vi "calc_trans.vi"(0 "Reference":T1, 3 "Input":T2) -> ()   [LabVIEW 2024]
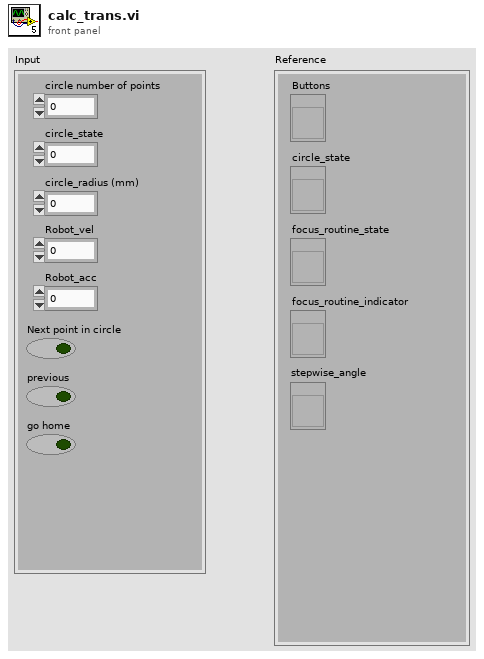
[diagram p1: front panel]
types:
  T1 = cluster{"Buttons":refnum<vi>, "circle_state":refnum<vi>, "focus_routine_state":refnum<vi>, "focus_routine_indicator":refnum<vi>, "stepwise_angle":refnum<vi>}
  T2 = cluster{"circle number of points":i8, "circle_state":i8, "circle_radius (mm)":dbl, "Robot_vel":dbl, "Robot_acc":dbl, "Next point in circle":bool, "previous":bool, "go home":bool}
  T3 = cluster{"Focus routine":bool, "Freedrive mode":bool, "Next point in circle":bool, "previous":bool, "go home":bool}
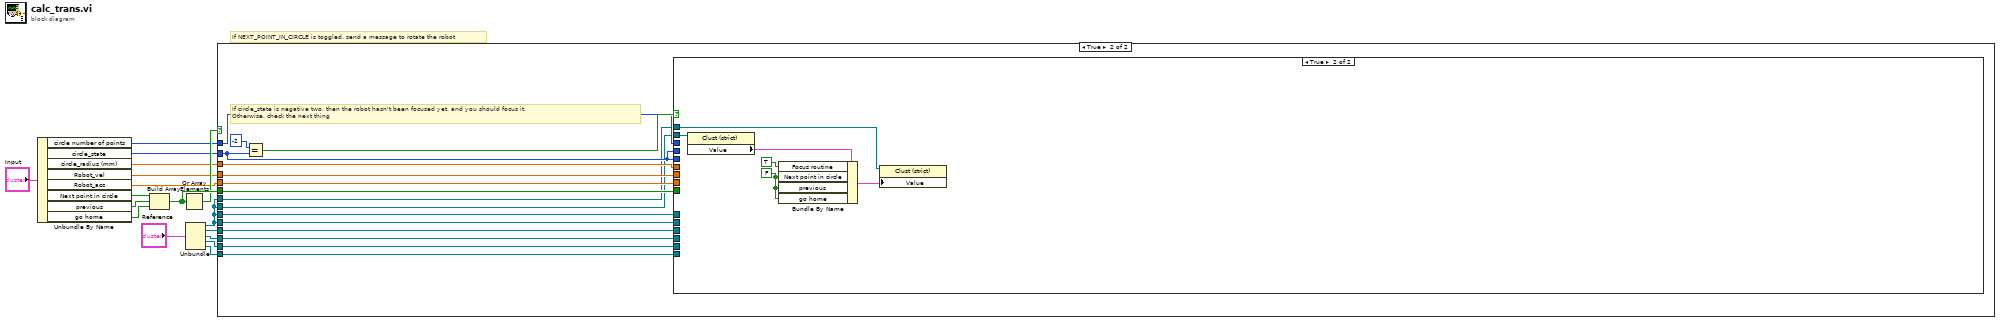
[diagram p0: block diagram]
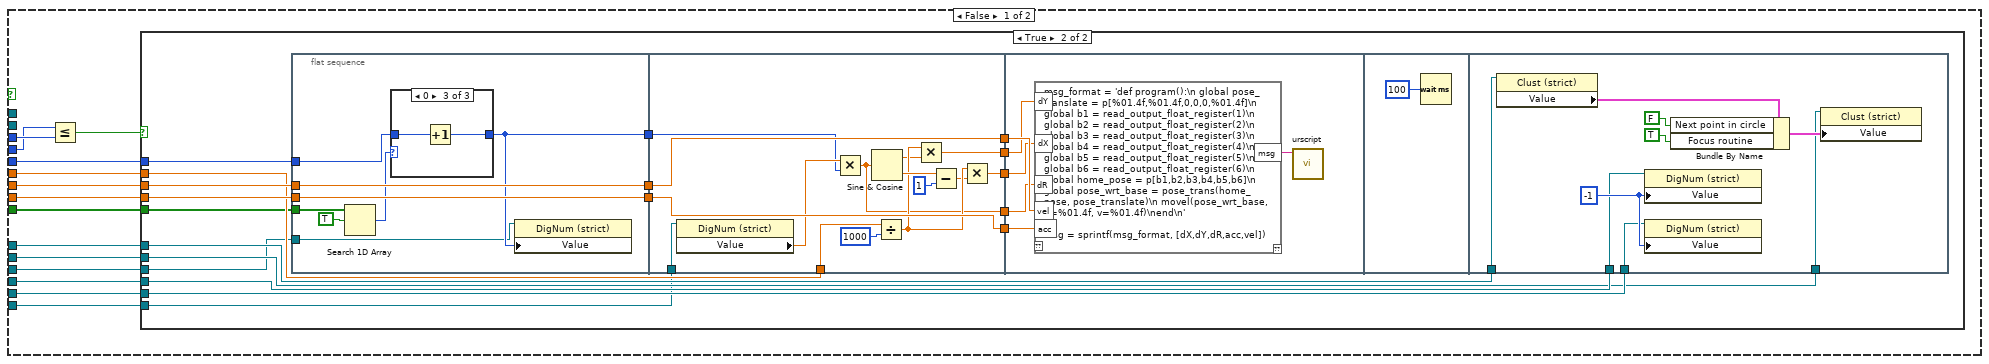
[diagram p3: hidden frame]
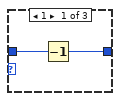
[diagram p5: hidden frame]
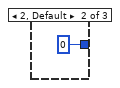
[diagram p6: hidden frame]
diagram:
  # "If NEXT_POINT_IN_CIRCLE is toggled, send a message to rotate the robot"
  n1 = Unbundle By Name("Input") -> ("circle number of points"=w14:i8, "circle_state"=w13:i8, "circle_radius (mm)"=w12:dbl, "Robot_vel"=w11:dbl, "Robot_acc"=w10:dbl, "Next point in circle"=w9:bool, "previous"=w7:bool, "go home"=w8:bool)
  n2 = Build Array(w9, w7, w8) -> (w17:bool[])
  n3 = Or Array Elements(Boolean array=w17) -> (logical OR=w16:bool)
  n4 = Unbundle("Reference") -> ("Buttons"=w5:refnum<vi>, "circle_state"=w4:refnum<vi>, "focus_routine_state"=w3:refnum<vi>, "focus_routine_indicator"=w2:refnum<vi>, "stepwise_angle"=w1:refnum<vi>)
  n5 = case shown="True" w16 {
    tunnel: w13 -> [_ w28]
    tunnel: w14 -> [_ w31]
    tunnel: w11 -> [_ w30]
    tunnel: w10 -> [_ w29]
    tunnel: w12 -> [_ w27]
    tunnel: w17 -> [_ w26]
    tunnel: w3 -> [_ w25]
    tunnel: w2 -> [_ w24]
    tunnel: w5 -> [_ w23]
    tunnel: w5 -> [_ w22]
    tunnel: w1 -> [_ w21]
    tunnel: w4 -> [_ w20]
    tunnel: w5 -> [_ w19]
    tunnel: w5 -> [_ w18]
    frame False {
    }
    frame True {
      # "If circle_state is negative two, then the robot hasn't been focused yet, and you should focus it.\nOtherwise, check the next thing"
      n6 = Equal?(x=-2, y=w28) -> (x = y?=w32:bool)
      n7 = case shown="True" w32 {
        tunnel: w31 -> [w43 _]
        tunnel: w28 -> [w42 _]
        tunnel: w30 -> [w47 _]
        tunnel: w29 -> [w46 _]
        tunnel: w28 -> [w45 _]
        tunnel: w27 -> [w44 _]
        tunnel: w26 -> [w40 _]
        tunnel: w25 -> [w39 _]
        tunnel: w24 -> [w38 _]
        tunnel: w23 -> [w37 _]
        tunnel: w22 -> [w36 _]
        tunnel: w21 -> [w35 _]
        tunnel: w20 -> [w34 _]
        tunnel: w19 -> [_ w112]
        tunnel: w18 -> [_ w111]
        frame False {
          n8 = Less Or Equal?(x=w42, y=w43) -> (x <= y?=w41:bool)
          n9 = case shown="True" w41 {
            tunnel: w47 -> [_ w66]
            tunnel: w46 -> [_ w65]
            tunnel: w45 -> [_ w56]
            tunnel: w44 -> [_ w57]
            tunnel: w40 -> [_ w54]
            tunnel: w39 -> [_ w53]
            tunnel: w38 -> [_ w52]
            tunnel: w37 -> [_ w51]
            tunnel: w36 -> [_ w50]
            tunnel: w35 -> [_ w49]
            tunnel: w34 -> [_ w48]
            frame False {
            }
            frame True {
              n10 = flat-sequence {
                tunnel: w56 -> [w72]
                tunnel: w65 -> [w73]
                tunnel: w66 -> [w74]
                tunnel: [w74] -> w59
                tunnel: [w73] -> w58
                tunnel: [w68] -> w55
                tunnel: w54 -> [w71]
                tunnel: w48 -> [w67]
                tunnel: [w94] -> w64
                tunnel: [w93] -> w63
                tunnel: [w82] -> w62
                tunnel: [w83] -> w61
                tunnel: [w84] -> w60
                tunnel: w59 -> [w94]
                tunnel: w58 -> [w93]
                tunnel: w57 -> [w86]
                tunnel: w55 -> [w81]
                tunnel: w49 -> [w80]
                tunnel: w64 -> [w100]
                tunnel: w63 -> [w99]
                tunnel: w62 -> [w98]
                tunnel: w61 -> [w97]
                tunnel: w60 -> [w96]
                tunnel: w53 -> [w105]
                tunnel: w52 -> [w104]
                tunnel: w51 -> [w103]
                tunnel: w50 -> [w102]
                frame #0 {
                  n11 = Search 1D Array(1D array=w71, element=TRUE) -> (index of element=w69:i32)  [unwired: 1 in]
                  n12 = case shown="0" w69 {
                    tunnel: w72 -> [w76 _ w79]
                    tunnel: [w75 0 w78] -> w68
                    frame 1 {
                      n13 = Decrement(x=w76) -> (x-1=w75:i8)
                    }
                    frame 2, Default {
                    }
                    frame 0 {
                      n14 = Increment(x=w79) -> (x+1=w78:i8)
                    }
                  }
                  n15 = property class="DigNum (strict)"(reference=w67, "Value"=w68) -> ()  [unwired: 1 in, 2 out]
                }
                frame #1 {
                  n16 = property class="DigNum (strict)"(reference=w80) -> ("Value"=w88:dbl)  [unwired: 1 in, 2 out]
                  n17 = Multiply(x=w88, y=w81) -> (x*y=w82:dbl)
                  n18 = Sine & Cosine(0:w82) -> (1:w89:dbl, 2:w92:dbl)
                  n19 = Divide(x=w86, y=1000) -> (x/y=w91:dbl)
                  n20 = Multiply(x=w91, y=w89) -> (x*y=w83:dbl)
                  n21 = Subtract(x=w92, y=1) -> (x-y=w90:dbl)
                  n22 = Multiply(x=w91, y=w90) -> (x*y=w84:dbl)
                }
                frame #2 {
                  n23 = script code="msg_format = 'def program():\\n global pose_translate = p[%01.4f,%01.4f,0,0,0,%01.4f]\\n global b1 = read_output_float_register(1)\\n global b2 = read_output_float_register(2)\\n global b3 = read_output_float_register(3)\\n global b4 = read_output_float_register(4)\\n global b5 = read_output_float_register(5)\\n global b6 = read_output_float_register(6)\\n global home_pose = p[b1,b2,b3,b4,b5,b6]\\n global pose_wrt_base = pose_trans(home_pose, pose_translate)\\n movel(pose_wrt_base, a=%01.4f, v=%01.4f)\\nend\\n'\n\nmsg = sprintf(msg_format, [dX,dY,dR,acc,vel])"("dX"=w96, "dY"=w97, "dR"=w98, "vel"=w100, "acc"=w99) -> ("msg"=w95:string)  [unwired: 1 in, 1 out]
                  n24 = call "urscript.vi"("String"=w95) -> ()  [unwired: 11 in]
                }
                frame #3 {
                  n25 = Wait (ms)(milliseconds to wait=100) -> ()  [unwired: 1 out]
                }
                frame #4 {
                  w110 = -1
                  n26 = property class="Clust (strict)"(reference=w102) -> ("Value"=w108:T3)  [unwired: 1 in, 2 out]
                  n27 = property class="DigNum (strict)"(reference=w105, "Value"=w110) -> ()  [unwired: 1 in, 2 out]
                  n28 = property class="DigNum (strict)"(reference=w104, "Value"=w110) -> ()  [unwired: 1 in, 2 out]
                  n29 = Bundle By Name(cluster=w108, "Next point in circle"=FALSE, "Focus routine"=TRUE) -> (w109:T3)
                  n30 = property class="Clust (strict)"(reference=w103, "Value"=w109) -> ()  [unwired: 1 in, 2 out]
                }
              }
            }
          }
        }
        frame True {
          w113 = FALSE
          n31 = property class="Clust (strict)"(reference=w111) -> ("Value"=w114:T3)  [unwired: 1 in, 2 out]
          n32 = Bundle By Name(cluster=w114, "Focus routine"=TRUE, "Next point in circle"=w113, "previous"=w113, "go home"=w113) -> (w115:T3)
          n33 = property class="Clust (strict)"(reference=w112, "Value"=w115) -> ()  [unwired: 1 in, 2 out]
        }
      }
    }
  }
